vi "Get_AnklePos.vi"(8 "error in (no error)":errorcluster, 11 "CAlexData in":refnum<class "CAlexData2.lvclass">) -> (0 "error out":errorcluster, 2 "AnklePos":dbl[][](array[numeric]), 3 "CAlexData out":refnum<class "CAlexData2.lvclass">)   [LabVIEW 2015, in "CAlexData2.lvclass"]
uses:
  CAlexData2.lvclass
  ExpData/ExpData.lvclass
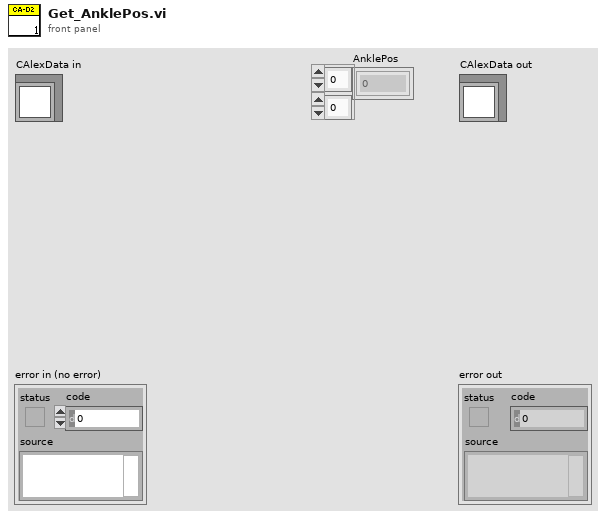
[diagram p1: front panel]
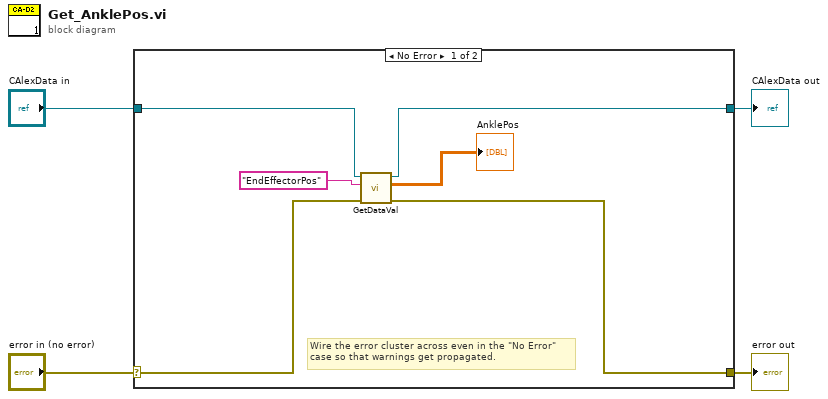
[diagram p0: block diagram]
diagram:
  n1 = case shown="No Error" "error in (no error)" {
    selector: "error in (no error)" -> [w8 w12]
    tunnel: [w7 w12] -> w3
    tunnel: [w9 w11] -> w1
    tunnel: "CAlexData in" -> [w10 w11]
    frame No Error {
      # "Wire the error cluster across even in the \"No Error\"\ncase so that warnings get propagated."
      n2 = call "GetDataVal.vi"("error in (no error)"=w8, "Name"="EndEffectorPos", "CarexMData in"=w10) -> ("error out"=w7:errorcluster, "Data"=→"AnklePos":dbl[][], "CarexMData out"=w9:refnum<class "CAlexData2.lvclass">)  [unwired: 5 in, 1 out]
    }
    frame Error {
    }
  }
  "error out" <- w3
  "CAlexData out" <- w1
